vi "test diagram.vi"() -> ()   [LabVIEW 2014]
uses:
  <vilib>/CANopenLib/CANOPEN.llb/CANopen Convert To Data [I16].vi
  <vilib>/CANopenLib/CANOPEN.llb/CANopen Fetch from Data [I16].vi
panel:
  out "Nächster ganzzahliger Wert":dbl
  out "signed 16-bit integer 2":i16
  in  "signed 16-bit integer":dbl
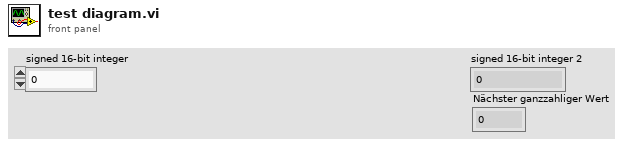
[diagram p1: front panel]
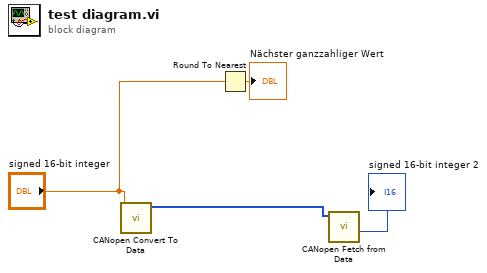
[diagram p0: block diagram]
diagram:
  n1 = call-poly <vilib>:"CANopen Convert To Data.vi"("signed 16-bit integer"="signed 16-bit integer") -> ("CANopen data out"=w4:u8[])  [unwired: 9 in, 1 out]
  n2 = Round To Nearest(number="signed 16-bit integer") -> (nearest integer value=→"Nächster ganzzahliger Wert":dbl)
  n3 = call-poly <vilib>:"CANopen Fetch from Data.vi"("CANopen data in"=w4) -> ("signed 16-bit integer"=→"signed 16-bit integer 2":i16)  [unwired: 8 in, 2 out]
